vi "libssh2_agent_userauth - invalid public key - no error 1097.vi"() -> ()   [LabVIEW 2013, in "libssh2_tests.lvlib"]
uses:
  libssh2_tests.lvlib
  libssh2/libssh2.lvlib
  libssh2/libssh2_init_default.vi
  <vilib>/addons/_JKI Toolkits/Caraya/classes/Test/Test.lvclass
  libssh2/libssh2_agent_publickey_refnum.ctl
panel:
  out "error out":errorcluster
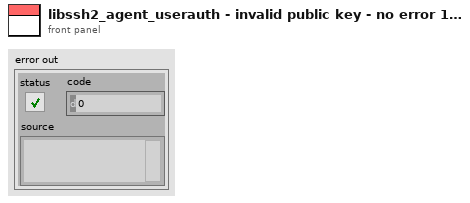
[diagram p1: front panel]
types:
  T1 = typedef "libssh2.lvlib/Session Refnum.ctl" = refnum<k1>
  T2 = typedef "libssh2.lvlib/Agent Refnum.ctl" = refnum<k1>
  T3 = typedef "libssh2.lvlib/libssh2_agent_publickey_refnum.ctl" = refnum<k1>
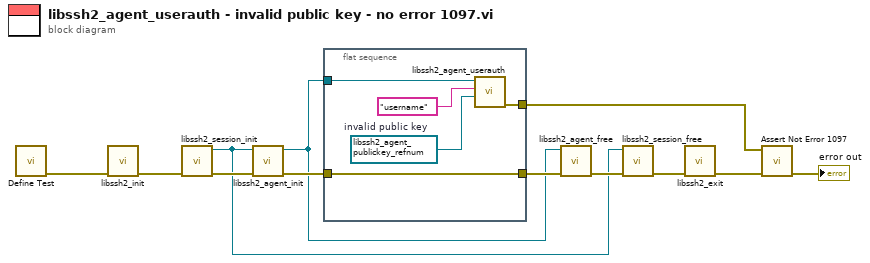
[diagram p0: block diagram]
diagram:
  n1 = call <vilib>:"Define Test.vi"() -> ("error out"=w12:errorcluster)  [unwired: 10 in, 1 out]
  n2 = call-poly "libssh2_init.vi"("error in (no error)"=w12) -> ("error out"=w10:errorcluster)  [unwired: 10 in]
  n3 = call "libssh2_session_init.vi"("error in (no error)"=w10) -> ("error out"=w6:errorcluster, "session"=w1:T1)  [unwired: 9 in]
  n4 = call "libssh2_agent_init.vi"("error in (no error)"=w6, "session"=w1) -> ("error out"=w5:errorcluster, "agent"=w3:T2)  [unwired: 8 in]
  n5 = flat-sequence {
    tunnel: [w17] -> w9
    tunnel: w5 -> [w17]
    tunnel: [w16] -> w8
    tunnel: w3 -> [w13]
    frame #0 {
      w15 = T3 refnum items=["publickey"]  # invalid public key
      n6 = call "libssh2_agent_userauth.vi"("public key"=w15, "username"="username", "agent"=w13) -> ("error out"=w16:errorcluster)  [unwired: 7 in, 1 out]
    }
  }
  n7 = call "libssh2_agent_free.vi"("error in (no error)"=w9, "agent"=w3) -> ("error out"=w4:errorcluster)  [unwired: 9 in]
  n8 = call "libssh2_session_free.vi"("error in (no error)"=w4, "session"=w1) -> ("error out"=w2:errorcluster)  [unwired: 9 in]
  n9 = call "libssh2_exit.vi"("error in (no error)"=w2) -> ("error out"=w11:errorcluster)  [unwired: 10 in]
  n10 = call "Assert Not Error 1097.vi"("error in (no error)"=w11, "actual value"=w8) -> ("error out"=→"error out":errorcluster)  [unwired: 9 in]
